vi "MotorConfig.vi"(8 "error in (no error)":errorcluster) -> (0 "error out":errorcluster, 3 "differential steering frame out":T1)   [LabVIEW 2017]
uses:
  <vilib>/robotics/Steering/Class Type Definitions/Differential Steering Frame.ctl
  <vilib>/robotics/Steering/Differential Steering Frame/NI_Robotics_Differential Steering Frame.lvclass
  <vilib>/robotics/Steering/Wheel/Wheel Parameters.ctl
  <vilib>/robotics/Steering/Wheel/Rotation Direction.ctl
  <vilib>/robotics/Steering/Fixed Wheel/NI_Robotics_Fixed Wheel.lvclass
  <vilib>/robotics/Steering/Wheel/NI_Robotics_Wheel.lvclass
  <vilib>/robotics/Steering/Class Type Definitions/NI_Robotics_Steering Class Types.lvlib
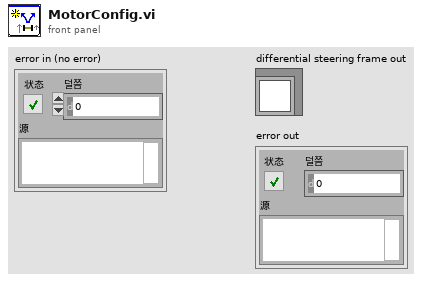
[diagram p1: front panel]
types:
  T1 = typedef "NI_Robotics_Steering Class Types.lvlib/Differential Steering Frame.ctl" = refnum<class "NI_Robotics_Differential Steering Frame.lvclass">
  T2 = typedef "NI_Robotics_Wheel.lvclass/Wheel Parameters.ctl" = cluster{"wheel radius":dbl, "gear ratio":dbl, "forward rotation direction":T3}
  T3 = typedef "NI_Robotics_Wheel.lvclass/Rotation Direction.ctl" = u16
  T4 = cluster{"fixed wheel out":refnum<class "NI_Robotics_Fixed Wheel.lvclass">, "fixed wheel out":refnum<class "NI_Robotics_Fixed Wheel.lvclass">}
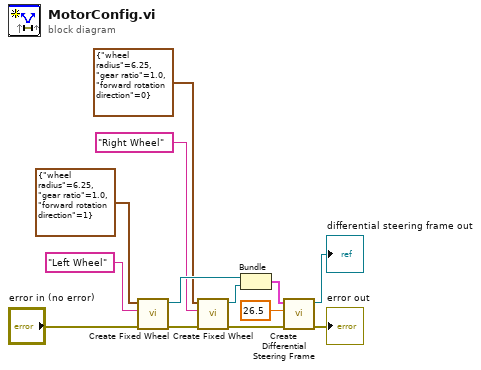
[diagram p0: block diagram]
diagram:
  n1 = call <vilib>:"Create Fixed Wheel.vi"("error in (no error)"="error in (no error)", "wheel name"="Left Wheel", "wheel parameters"=T2 {"wheel radius"=6.25, "gear ratio"=1.0, "forward rotation direction"=1}) -> ("error out"=w5:errorcluster, "fixed wheel out"=w8:refnum<class "NI_Robotics_Fixed Wheel.lvclass">)  [unwired: 7 in]
  n2 = call <vilib>:"Create Fixed Wheel.vi"("error in (no error)"=w5, "wheel name"="Right Wheel", "wheel parameters"=T2 {"wheel radius"=6.25, "gear ratio"=1.0, "forward rotation direction"=0}) -> ("error out"=w3:errorcluster, "fixed wheel out"=w4:refnum<class "NI_Robotics_Fixed Wheel.lvclass">)  [unwired: 7 in]
  n3 = Bundle("fixed wheel out"=w8, "fixed wheel out"=w4) -> (w12:T4)  [unwired: 1 in]
  n4 = call <vilib>:"Create Differential Steering Frame.vi"("error in (no error)"=w3, "wheel separation"=26.5, "wheels"=w12) -> ("error out"=→"error out":errorcluster, "differential steering frame out"=→"differential steering frame out":refnum<class "NI_Robotics_Differential Steering Frame.lvclass">)  [unwired: 7 in]
